vi "Configuration.vi"() -> (0 "error out":errorcluster, 2 "Configuration":T1)   [LabVIEW 2013]
uses:
  <vilib>/Utility/config.llb/Read Key (Boolean).vi
  <vilib>/Utility/config.llb/Read Key (String).vi
  <vilib>/Utility/config.llb/Read Key (Path).vi
  <vilib>/Utility/config.llb/Read Key (I32).vi
  <vilib>/Utility/config.llb/Read Key (Double).vi
  <vilib>/Utility/config.llb/NI_LVConfig.lvlib
panel:
  in  "configuration file path":path
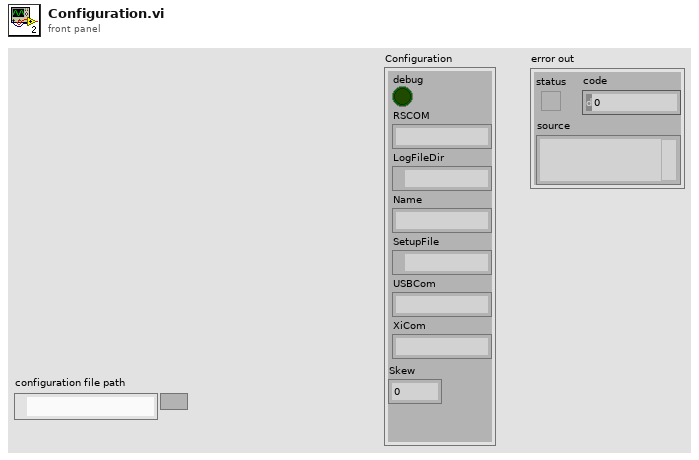
[diagram p1: front panel]
types:
  T1 = cluster{"debug":bool, "RSCOM":string, "LogFileDir":path, "Name":string, "SetupFile":path, "USBCom":string, "XiCom":string, "Skew":dbl}
  T2 = typedef "NI_LVConfig.lvlib/Config Data RefNum.ctl" = refnum<k1>
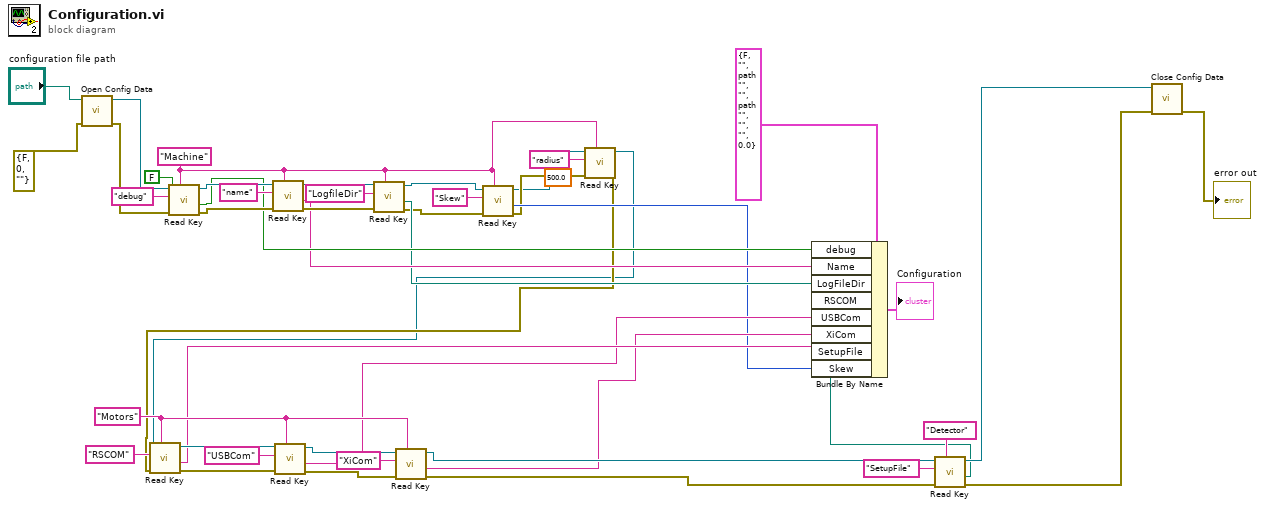
[diagram p0: block diagram]
diagram:
  w34 = "Motors" ("section")
  w6 = "Machine" ("section")
  n1 = call <vilib>:"Open Config Data.vi"("error in (no error)"=errorcluster {"status"=FALSE, "code"=0, "source"=""}, "configuration file path"="configuration file path") -> ("error out"=w44:errorcluster, "refnum"=w38:T2)  [unwired: 7 in, 1 out]
  n2 = call-poly <vilib>:"Read Key.vi"("section"=w6, "error in (no error)"=w44, "default value"=FALSE, "key"="debug", "refnum"=w38) -> ("error out"=w43:errorcluster, "value"=w32:bool, "refnum out"=w37:T2)  [unwired: 3 in, 1 out]
  n3 = call-poly <vilib>:"Read Key.vi"("section"=w6, "error in (no error)"=w43, "key"="name", "refnum"=w37) -> ("error out"=w42:errorcluster, "value"=w31:string, "refnum out"=w36:T2)  [unwired: 4 in, 1 out]
  n4 = call-poly <vilib>:"Read Key.vi"("section"=w6, "error in (no error)"=w42, "key"="LogfileDir", "refnum"=w36) -> ("error out"=w12:errorcluster, "value"=w30:path, "refnum out"=w11:T2)  [unwired: 4 in, 1 out]
  n5 = call-poly <vilib>:"Read Key.vi"("section"=w6, "error in (no error)"=w12, "key"="Skew", "refnum"=w11) -> ("error out"=w5:errorcluster, "value"=w10:i32, "refnum out"=w2:T2)  [unwired: 4 in, 1 out]
  n6 = call-poly <vilib>:"Read Key.vi"("section"=w6, "error in (no error)"=w5, "default value"=500.0, "key"="radius", "refnum"=w2) -> ("error out"=w4:errorcluster, "refnum out"=w3:T2)  [unwired: 3 in, 2 out]
  n7 = call-poly <vilib>:"Read Key.vi"("section"=w34, "error in (no error)"=w4, "key"="RSCOM", "refnum"=w3) -> ("error out"=w24:errorcluster, "value"=w17:string, "refnum out"=w29:T2)  [unwired: 4 in, 1 out]
  n8 = call-poly <vilib>:"Read Key.vi"("section"=w34, "error in (no error)"=w24, "key"="USBCom", "refnum"=w29) -> ("error out"=w23:errorcluster, "value"=w16:string, "refnum out"=w28:T2)  [unwired: 4 in, 1 out]
  n9 = call-poly <vilib>:"Read Key.vi"("section"=w34, "error in (no error)"=w23, "key"="XiCom", "refnum"=w28) -> ("error out"=w22:errorcluster, "value"=w15:string, "refnum out"=w27:T2)  [unwired: 4 in, 1 out]
  n10 = call-poly <vilib>:"Read Key.vi"("section"="Detector", "error in (no error)"=w22, "key"="SetupFile", "refnum"=w27) -> ("error out"=w25:errorcluster, "value"=w14:path, "refnum out"=w26:T2)  [unwired: 4 in, 1 out]
  n11 = Bundle By Name(cluster=T1 {"debug"=FALSE, "RSCOM"="", "LogFileDir"=path "", "Name"="", "SetupFile"=path "", "USBCom"="", "XiCom"="", "Skew"=0.0} ("Configuration"), "debug"=w32, "Name"=w31, "LogFileDir"=w30, "RSCOM"=w17, "USBCom"=w16, "XiCom"=w15, "SetupFile"=w14, "Skew"=w10) -> (→"Configuration":T1)
  n12 = call <vilib>:"Close Config Data.vi"("error in (no error)"=w25, "refnum"=w26) -> ("error out"=→"error out":errorcluster)  [unwired: 8 in, 1 out]
